vi "WriteText.vi"(8 "error in (no error)":errorcluster, 9 "Appending":bool=TRUE, 10 "Input Text":string, 11 "File Path":path=path "F:/Data_Min") -> (0 "error out":errorcluster)   [LabVIEW 2018]
panel:
  # "WriteText: Write text/strings to txt file.\n1) If there is no existing file, the VI creates one;\n2) if Appending text to file is checked, the VI opens the exsiting file and appends the text/strings to the file; Otherwise the VI creates a new file and replaces the exsiting one."
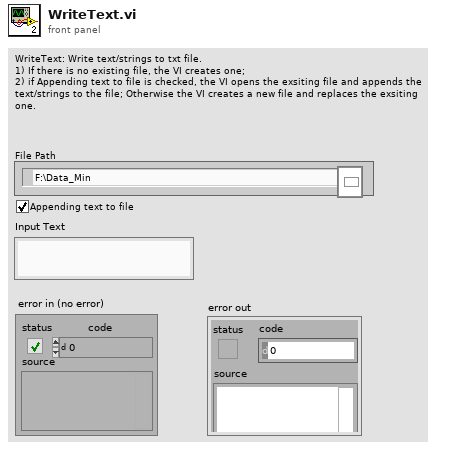
[diagram p1: front panel]
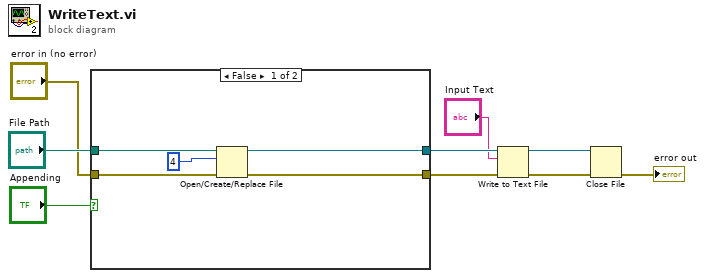
[diagram p0: block diagram]
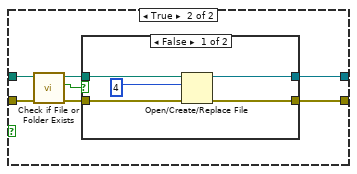
[diagram p2: hidden frame]
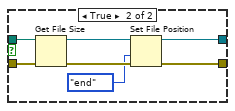
[diagram p3: hidden frame]
diagram:
  n1 = case shown="False" "Appending" {
    tunnel: "File Path" -> [w13 w20]
    tunnel: [w12 w17] -> w6
    tunnel: [w11 w18] -> w5
    tunnel: "error in (no error)" -> [w10 w16]
    frame False {
      n2 = Open/Create/Replace File(file path (use dialog)=w13, error in=w10, operation (0:open)=4) -> (refnum out=w11:refnum<file>, error out=w12:errorcluster)  [unwired: 3 in, 1 out]
    }
    frame True {
      n3 = call <vilib>:"Check if File or Folder Exists.vi"("error in (no error)"=w16, "path"=w20) -> ("error out"=w15:errorcluster, "file or folder exists?"=w21:bool, "dup path"=w19:path)  [unwired: 7 in]
      n4 = case shown="False" w21 {
        tunnel: w19 -> [w25 w33]
        tunnel: [w24 w31] -> w18
        tunnel: [w23 w30] -> w17
        tunnel: w15 -> [w22 w27]
        frame False {
          n5 = Open/Create/Replace File(file path (use dialog)=w25, error in=w22, operation (0:open)=4) -> (refnum out=w24:refnum<file>, error out=w23:errorcluster)  [unwired: 3 in, 1 out]
        }
        frame True {
          n6 = Get File Size(file=w33, error in=w27) -> (refnum out=w32:refnum<file>, 0:w29:errorcluster)  [unwired: 1 out]
          n7 = Set File Position(refnum=w32, from (0:start)=enum16{"start", "end", "current"}."end", error in=w29) -> (refnum out=w31:refnum<file>, error out=w30:errorcluster)  [unwired: 1 in]
        }
      }
    }
  }
  n8 = Write to Text File(file (use dialog)=w5, text="Input Text", error in=w6) -> (refnum out=w3:refnum<file>, error out=w2:errorcluster)  [unwired: 1 in, 1 out]
  n9 = Close File(refnum=w3, error in=w2) -> (error out=→"error out":errorcluster)  [unwired: 1 out]
